vi "PUT Y Position Set-point.vi"(0 "Y Position Set-point":dbl) -> ()   [LabVIEW 2013]
uses:
  Action.ctl
  Set Points FGV Selector.ctl
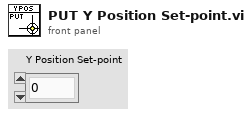
[diagram p1: front panel]
types:
  T1 = typedef "Set Points FGV Selector.ctl" = enum16{"X Position", "Y Position", "Z Position", "Z Scan"}
  T2 = typedef "Action.ctl" = enum16{"GET", "PUT", "DELETE"}
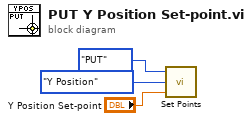
[diagram p0: block diagram]
diagram:
  n1 = call "Set Points.vi"("Input"="Y Position Set-point", "Set Points FGV Selector"=Set_Points_FGV_Selector."Y Position", "Action"=Action."PUT") -> ()  [unwired: 1 out]
